vi "Terminate.vi"(8 "error in (no error)":errorcluster, 10 "Message in":refnum<class "TerminateMessage.lvclass">, 11 "Cobolt in":refnum<class "Cobolt.lvclass">) -> (0 "error out":errorcluster, 3 "Cobolt out":refnum<class "Cobolt.lvclass">)   [LabVIEW 2012, in "Cobolt.lvclass"]
doc: "This member function is called when the statemachine in the run.vi receives an 'terminate' command. It closes the RabbitMQ connection. \n\nOverride this member function in your derived class to release all previously acquired resources (but don't forget to call the parent method). If your component has subcomponents, they count as resources, and you have to release them by calling their own terminate functions."
uses:
  Cobolt.lvclass
  <vilib>/Distrio/Murmex/TerminateMessage/TerminateMessage.lvclass
  Cobolt.lvclass/Cobolt.ctl
  <vilib>/Distrio/Murmex/Murmex/Murmex.lvclass
panel:
  # "This method is called when the TERMINATE\ntrigger is sent. \n\nOverride this method when your component needs to\nrespond to this trigger. \n\nCall parent for proper implementation"
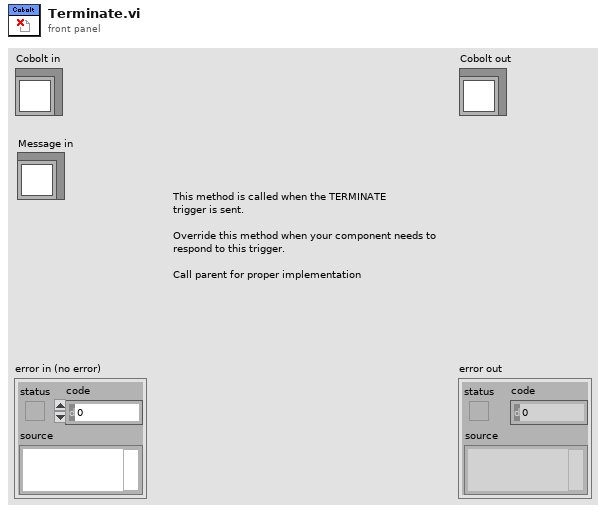
[diagram p1: front panel]
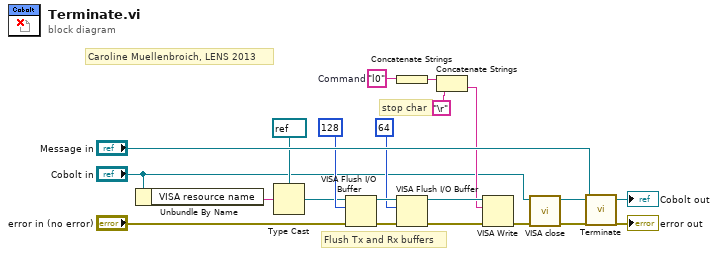
[diagram p0: block diagram]
diagram:
  w16 = "l0"  # Command
  # "stop char"
  # "Flush Tx and Rx buffers"
  # "Caroline Muellenbroich, LENS 2013"
  n1 = Unbundle By Name("Cobolt in") -> ("VISA resource name"=w5:string)
  n2 = Type Cast(type=refnum<visa-resource-name> refnum ("VISA resource name"), x=w5) -> (*(type *) &x=w9:refnum<visa-resource-name>)
  n3 = VISA Flush I/O Buffer(VISA resource name=w9, mask (16)=u16 128, error in (no error)="error in (no error)") -> (VISA resource name out=w14:refnum<visa-resource-name>, error out=w15:errorcluster)
  n4 = Concatenate Strings(w16) -> (w2:string)
  n5 = VISA Flush I/O Buffer(VISA resource name=w14, mask (16)=u16 64, error in (no error)=w15) -> (VISA resource name out=w10:refnum<visa-resource-name>, error out=w11:errorcluster)
  n6 = Concatenate Strings(w2, "\r") -> (w7:string)
  n7 = VISA Write(VISA resource name=w10, write buffer=w7, error in (no error)=w11) -> (error out=w1:errorcluster)  [unwired: 2 out]
  n8 = call-dynamic "VISA close.vi"("error in (no error)"=w1, "Cobolt in"="Cobolt in") -> ("error out"=w18:errorcluster, "Cobolt out"=w17:refnum<class "Cobolt.lvclass">)  [unwired: 8 in]
  n9 = call-parent "Terminate.vi"("error in (no error)"=w18, "Message in"="Message in", "Murmex in"=w17) -> ("error out"=→"error out":errorcluster, "Murmex out"=→"Cobolt out":refnum<class "Cobolt.lvclass">)  [unwired: 7 in]
